vi "ConnectRobot.vi"(8 "error in (no error)":errorcluster caption="Fehler (Eingang, kein Fehler)", 11 "Moveo Eingang":refnum<class "Moveo.lvclass">) -> (0 "error out":errorcluster caption="Fehler (Ausgang)", 3 "Moveo Ausgang":refnum<class "Moveo.lvclass">)   [LabVIEW 2019, in "Moveo.lvclass"]
uses:
  Moveo.lvclass
  Moveo.lvclass/Moveo.ctl
  MoveoSerialClass/MoveoSerial.lvclass
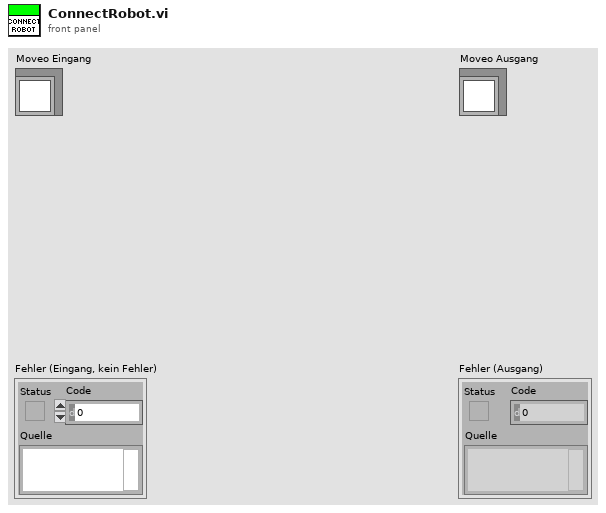
[diagram p1: front panel]
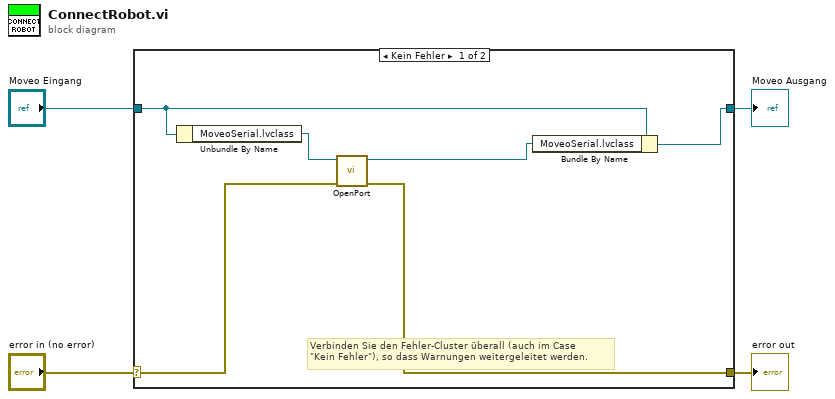
[diagram p0: block diagram]
diagram:
  n1 = case shown="Kein Fehler" "error in (no error)" {
    selector: "error in (no error)" -> [w9 w12]
    tunnel: [w8 w12] -> w3
    tunnel: [w6 w11] -> w1
    tunnel: "Moveo Eingang" -> [w7 w11]
    frame No Error {
      # "Verbinden Sie den Fehler-Cluster überall (auch im Case\n\"Kein Fehler\"), so dass Warnungen weitergeleitet werden."
      n2 = Unbundle By Name(w7) -> ("MoveoSerial.lvclass"=w10:refnum<class "MoveoSerial.lvclass">)
      n3 = call-dynamic "OpenPort.vi"("error in (no error)"=w9, "MoveoSerial Eingang"=w10) -> ("error out"=w8:errorcluster, "MoveoSerial Ausgang"=w5:refnum<class "MoveoSerial.lvclass">)  [unwired: 8 in]
      n4 = Bundle By Name(cluster=w7, "MoveoSerial.lvclass"=w5) -> (w6:refnum<class "Moveo.lvclass">)
    }
    frame Error {
    }
  }
  "error out" <- w3
  "Moveo Ausgang" <- w1
